vi "Parse Scripts.vi"(11 "Array":dbl[][](array[numeric])) -> ()   [LabVIEW 2015]
uses:
  Common Code/Auton Command Cluster.ctl
  Robot Global Data.vi
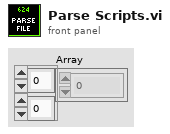
[diagram p1: front panel]
types:
  T1 = typedef "Auton Command Cluster.ctl" = cluster{"Command ID":i32, "maxTime":dbl, "Y Distance":dbl, "Heading":dbl, "Throttle":dbl, "Async":dbl, "Velocity":dbl, "Acceleration":dbl, "To":dbl, "Condition":dbl, "Shot Type":dbl, "Left RPM":dbl, "Override RPM":i32, "Override Angle":i32, "Right RPM":dbl, "Angle":dbl, "Intake Mode":i32, "Intake Cmd":i32, "Intake O":i32, "Eject O":i32, "Angle O":i32, "Arm O":i32, "Intake Speed":dbl, "Eject Speed":dbl, "Arm Angle":dbl, "Arm Speed":dbl, "Intake?":i32, "Eject?":i32, "Left":dbl, "Right":dbl, "Pivot Speed":dbl, "Y Dist":dbl, "Position":dbl, "Desired Position":i32, "Shooter Mode":dbl, "Shooter Command":dbl, "Shoot?":i32, "Shoot mode":i32}
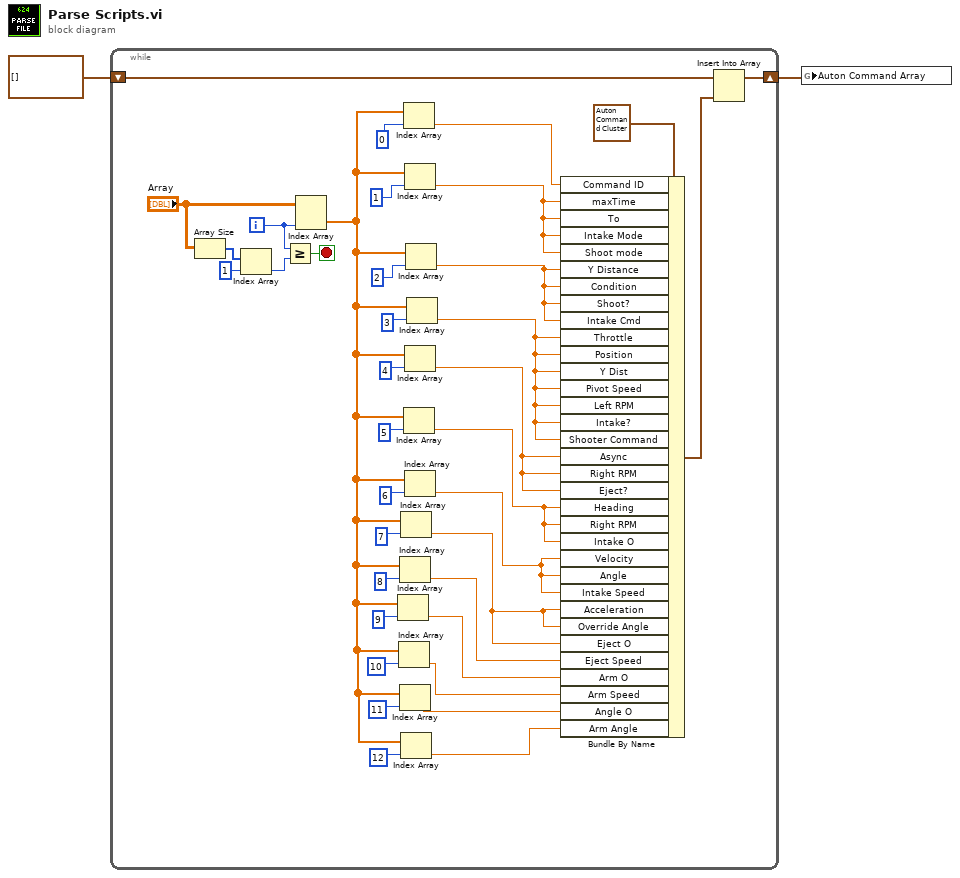
[diagram p0: block diagram]
diagram:
  n1 = while {
    shift-right: [w22] -> w1
    shift-left: T1[] [] -> [w23]
    i -> [w34]
    stop <- w32 stop-if-true
    n2 = Array Size(array="Array") -> (size(s)=w30:i32[])
    n3 = Index Array(array=w30, index=1) -> (element=w28:i32)
    n4 = Greater Or Equal?(x=w34, y=w28) -> (x >= y?=w32:bool)
    n5 = Index Array(array="Array", index (col)=w34) -> (element=w5:dbl[])  [unwired: 1 in]
    n6 = Index Array(array=w5, index=9) -> (element=w14:dbl)
    n7 = Index Array(array=w5, index=10) -> (element=w12:dbl)
    n8 = Index Array(array=w5, index=8) -> (element=w16:dbl)
    n9 = Index Array(array=w5, index=11) -> (element=w10:dbl)
    n10 = Index Array(array=w5, index=7) -> (element=w6:dbl)
    n11 = Index Array(array=w5, index=12) -> (element=w8:dbl)
    n12 = Index Array(array=w5, index=0) -> (element=w26:dbl)
    n13 = Index Array(array=w5, index=5) -> (element=w19:dbl)
    n14 = Index Array(array=w5, index=1) -> (element=w4:dbl)
    n15 = Index Array(array=w5, index=4) -> (element=w20:dbl)
    n16 = Index Array(array=w5, index=6) -> (element=w18:dbl)
    n17 = Index Array(array=w5, index=2) -> (element=w7:dbl)
    n18 = Index Array(array=w5, index=3) -> (element=w3:dbl)
    n19 = Bundle By Name(cluster=T1 {"Command ID"=0, "maxTime"=0.0, "Y Distance"=0.0, "Heading"=0.0, "Throttle"=0.0, "Async"=0.0, "Velocity"=0.0, "Acceleration"=0.0, "To"=0.0, "Condition"=0.0, "Shot Type"=0.0, "Left RPM"=0.0, "Override RPM"=0, "Override Angle"=0, "Right RPM"=0.0, "Angle"=0.0, "Intake Mode"=0, "Intake Cmd"=0, "Intake O"=0, "Eject O"=0, "Angle O"=0, "Arm O"=0, "Intake Speed"=0.0, "Eject Speed"=0.0, "Arm Angle"=0.0, "Arm Speed"=0.0, "Intake?"=0, "Eject?"=0, "Left"=0.0, "Right"=0.0, "Pivot Speed"=0.0, "Y Dist"=0.0, "Position"=0.0, "Desired Position"=0, "Shooter Mode"=0.0, "Shooter Command"=0.0, "Shoot?"=0, "Shoot mode"=0} ("Auton Command Cluster"), "Command ID"=w26, "maxTime"=w4, "To"=w4, "Intake Mode"=w4, "Shoot mode"=w4, "Y Distance"=w7, "Condition"=w7, "Shoot?"=w7, "Intake Cmd"=w7, "Throttle"=w3, "Position"=w3, "Y Dist"=w3, "Pivot Speed"=w3, "Left RPM"=w3, "Intake?"=w3, "Shooter Command"=w3, "Async"=w20, "Right RPM"=w20, "Eject?"=w20, "Heading"=w19, "Right RPM"=w19, "Intake O"=w19, "Velocity"=w18, "Angle"=w18, "Intake Speed"=w18, "Acceleration"=w6, "Override Angle"=w6, "Eject O"=w6, "Eject Speed"=w16, "Arm O"=w14, "Arm Speed"=w12, "Angle O"=w10, "Arm Angle"=w8) -> (w21:T1)
    n20 = Insert Into Array(array=w23, new element=w21) -> (w22:T1[])  [unwired: 1 in]
  }
  n21 = global write "Robot Global Data.vi" "Auton Command Array"(w1) -> ()
